vi "reference.vi"(9 "imin constant (10)":dbl=10.0 format="%.2f", 10 "GPIB":string="18") -> (0 "canceled":bool, 1 "Amax":dbl[](array[numeric])=[1.4910673946532929, 1.6585837154070626, 1.7446058754142388, 1.808885867359812, 1.8820632464916343, 1.9639766099966056, 2.0382226383687185, 2.089414045842038, 2.105029640404689, 2.0885577699852065, 2.0571333672490866, 2.027508616078245, 2.015359755409214, 2.0257112906258596, 2.0595634179012676, 2.1100473453298383, 2.172833443035523, 2.234615975589444, 2.2871273786148105, 2.3224260524059526, 2.3363376339055857, 2.331182240765136, 2.314328676539224, 2.289898733886235, 2.2678754193188975, 2.2505151462951534, 2.242292904982931, 2.24398006574108, 2.2563785464280435, 2.27769858497494, 2.3057403402615764, 2.3370197526004075, 2.366945663852573, 2.3897701311083424, 2.4032921451582543, 2.40229406080999, 2.3862474121289834, 2.3547632303177037, 2.315886415708487, 2.2697907104438184, 2.2262905051834165, 2.187520720836463, 2.160711571967675, 2.14674801363064, 2.144452774972763, 2.153387979331808, 2.171612381536747, 2.1975010961432586, 2.2293259691913074, 2.2656195831538843, 2.3051814883832087, 2.3454913564746462, 2.3821233506183246, 2.4127964287165433, 2.4358762045887516, 2.4497868469857735, 2.4546009770977615, 2.4515101179343155, 2.4418223425174155, 2.426641367561445, 2.406916405977408, 2.3842458578199786, 2.362557866554489, 2.33933415602267, 2.3189810644947233, 2.300073495267144, 2.2845660772669736, 2.2714233677435813, 2.26150315158433, 2.253967663414962, 2.2510539021873077, 2.2506151469906333, 2.2525617862063294, 2.2579664095081773, 2.2654805602840473, 2.2745273043960443, 2.28510928212571, 2.296358004741391, 2.309161557904644, 2.3221779313849757, 2.3315082762863897, 2.3426595041391187, 2.3506375453397452, 2.3588101724585626, 2.3636890556226735, 2.3664229572259727, 2.3670948931236584, 2.333326340403454, 2.224794544652323, 2.280031744138702, 2.2816718335664525, 2.270259475526624, 2.26226356693396, 2.2632572270140665, 2.2654310668267126, 2.271051261492347, 2.252318932941653, 2.2465502794425976, 2.235677394469935, 2.249345136353329, 2.2270635923428257, 2.230806428468883, 2.249200804113696, 2.2253609803726593, 2.2477278329097232, 2.2421934558224543, 2.21325471004923, 2.213995616368085, 2.2355284469075487, 2.1967287226232872, 2.2059618230596336, 2.2089248310802643, 2.233455559096529, 2.2098365950696555, 2.2121876044039577, 2.229118455328952, 2.297850204978715, 2.290123688274307, 2.251689310911409, 2.2801228963023075, 2.315594633653461, 2.2778841422402, 2.2936276917660194, 2.281533313857376, 2.293232136279035, 2.298328988073495, 2.3684356541018055, 2.3648510520076926, 2.362067585727399, 2.3472128864048627, 2.344902908055406, 2.322053817695566, 2.3018977171952084, 2.309502414966703, 2.341238602698547, 2.3314272965207428, 2.281081114278017, 2.3288686738529263, 2.336181456081918, 2.261833620575751, 2.183215731491115, 2.177997963096566, 2.21197440141396, 2.212879792163401, 2.195456833628169, 2.2016155823139427, 2.2219355998280053, 2.2220918864542596, 2.5689054149828787, 2.208387603795154, 2.1666106622894317, 2.126780577012009, 2.1150777166595804, 2.0993352776859577, 2.0773679052841567, 2.090610707828407, 2.0946108630321367, 2.0626571802255635, 2.043283665570575, 2.006123606211854, 1.9866821797795053, 1.9793662423961613, 1.9486134383505207, 1.9236584217933062, 1.8991636414772188, 1.8864907251724818, 1.852601969338235, 1.847449262499173, 1.8450980400142565, 1.8481891169913987, 1.8517535290295353, 1.843730965112092, 1.9172954009456893, 1.8857003801283296, 1.9035240644712623, 1.9124293202224247, 1.9338970927268733, 1.9433955765089543, 1.9029813997975025, 1.975059396468232, 1.902764143924086, 1.9264402033377668, 1.9214835839687896, 1.9399184203690565, 1.905364068766892, 1.9486085498764363, 1.959608944863131, 1.9838967913263057, 2.00337435401975, 2.1681437754959583, 2.370476079544294, 2.434505032502073, 2.513031053176271, 2.501251021855857, 2.6030360562505215, 2.553057325316767, 2.6755217206077972, 2.4904080015060113, 2.5658950220301104, 2.566814463504501, 2.4194286609338724, 2.452277233126352, 2.549567233145539, 2.489508491577916, 2.466036775232349, 2.5291222348209623, 2.5165882528051435, 2.5152378253184304, 2.2831654904677503, 2.1027766148834415, 2.2945103147339774, 2.278296208091274, 2.2947747522184434, 2.257102332659164, 2.1926232000129464, 2.1866738674997452, 2.1486674240110664, 2.1793794178817567, 2.081707270097349, 2.0340666785975605, 2.017705140697976, 1.918240090221415, 1.8567288903828827, 1.8983960459300089, 1.8564872128686305, 1.803320523578754, 1.7109631189952759, 1.7223047868743275, 1.6916207084305435, 1.770991846672562, 1.8018220229225788, 1.8637985386805003, 1.6497241859295224, 2.4798055677093918, 1.8810421081934057, 1.9936125579388904, 1.7551198989199506, 1.6860908247574418, 1.670255132771604, 1.6022662322285295, 1.646207612206685, 1.8161086707399037, 1.682686478249768, 1.6551384348113822, 1.732562619289829, 1.8138477542288545, 1.7537438789213702, 1.8034571156484138, 1.9565573917856787, 1.8325089127062364, 1.7867514221455612, 1.8590181438888942, 1.8106289836371174, 1.7455432019980242, 1.8923172607224805, 1.7453871213200087, 1.7158362751649936, 1.717670503002262, 1.681612038904928, 1.9141315126308938, 1.7541877393996606, 1.72965066833592, 1.8286598965353196, 1.793923026734563, 1.7128264134251168, 1.777716738609626, 1.7576996250877386, 1.7315887651867385, 1.8689969024871353, 1.8407332346118066, 1.8972971220594963, 1.9706257766882944, 1.9689496809813425, 1.9907826918031377, 1.9205407165024797, 1.9384196457931928, 1.8095597146352675, 1.7610252517113727, 1.7540423867854362, 1.823474229170301, 1.8949858218973574, 1.9153998352122696, 1.9240724299103626, 1.9669860251179379, 2.1140101617034617, 2.0889825806046582, 2.0437590536641457, 2.011316643366872, 2.049838000622583, 1.8634418286137089, 2.044069150468914, 1.9808211666443354, 1.8472023639809236, 1.721645766289746, 1.7299742856995555, 1.8672317145188941, 1.8999298827278643, 1.8678209080455728, 1.7734865759276401, 1.8046845149069402, 1.8242625467907634, 1.7199938263676038, 1.789150434745198, 1.8715729355458788, 1.6698652146556314, 1.6812412373755872, 1.665027217492617, 1.6261349786353885, 1.6803355134145632, 1.7762652182681096, 1.6748611407378116, 1.578180609627778, 1.5795549604009986, 1.611925011653304, 1.54282542695918, 1.5206145218782359] format="%.2f", 2 "IR":dbl[](array[numeric])=[309.78999999999996, 455.5999999999999, 555.4000000000001, 644.0, 762.19, 920.3999999999999, 1092.0, 1228.6100000000001, 1273.5900000000001, 1226.19, 1140.6, 1065.39, 1036.0, 1060.99, 1147.0, 1288.3899999999999, 1488.79, 1716.3899999999999, 1936.9899999999998, 2101.0, 2169.3900000000003, 2143.79, 2062.19, 1949.3899999999999, 1853.0, 1780.3899999999999, 1747.0, 1753.8000000000002, 1804.5900000000001, 1895.3899999999999, 2021.81, 2172.8, 2327.7999999999997, 2453.41, 2531.0, 2525.19, 2433.59, 2263.41, 2069.6, 1861.19, 1683.8000000000002, 1540.0, 1447.81, 1402.0, 1394.6100000000001, 1423.6, 1484.6100000000001, 1575.8000000000002, 1695.6100000000001, 1843.4, 2019.21, 2215.6, 2410.59, 2587.0, 2728.2, 2817.0, 2848.4, 2828.2, 2765.81, 2670.8, 2552.21, 2422.4, 2304.4, 2184.41, 2084.4, 1995.6, 1925.6, 1868.1999999999998, 1826.0099999999998, 1794.6, 1782.6, 1780.8000000000002, 1788.8000000000002, 1811.1999999999998, 1842.81, 1881.6, 1928.0099999999998, 1978.6, 2037.8000000000002, 2099.8, 2145.4, 2201.2, 2242.01, 2284.6, 2310.41, 2325.0, 2328.6, 2154.4, 1678.0099999999998, 1905.6, 1912.81, 1863.1999999999998, 1829.21, 1833.4, 1842.6, 1866.6, 1787.8000000000002, 1764.21, 1720.5900000000001, 1775.6, 1686.8000000000002, 1701.4, 1775.0099999999998, 1680.1999999999998, 1769.0, 1746.6, 1634.0099999999998, 1636.8000000000002, 1720.0, 1573.0, 1606.8000000000002, 1617.8000000000002, 1711.81, 1621.1999999999998, 1630.0, 1694.8000000000002, 1985.4099999999999, 1950.4, 1785.21, 1906.0, 2068.21, 1896.1999999999998, 1966.2000000000003, 1912.1999999999998, 1964.4099999999999, 1987.6, 2335.8, 2316.6, 2301.8, 2224.4, 2212.6, 2099.2, 2004.0000000000002, 2039.4, 2194.0099999999998, 2145.0, 1910.21, 2132.4, 2168.61, 1827.4, 1524.81, 1506.6, 1629.1999999999998, 1632.6, 1568.3999999999999, 1590.8000000000002, 1667.0, 1667.6, 3706.0, 1615.8000000000002, 1467.6099999999997, 1339.0, 1303.4, 1257.0, 1195.0, 1232.0, 1243.4, 1155.1999999999998, 1104.8000000000002, 1014.2, 969.8000000000001, 953.5999999999999, 888.4099999999999, 838.8, 792.8, 770.0, 712.1999999999999, 703.8, 699.9999999999999, 705.0, 710.8100000000001, 697.8, 826.5999999999999, 768.5999999999999, 800.8000000000001, 817.3900000000001, 858.81, 877.8, 799.8, 944.19, 799.4000000000001, 844.19, 834.6099999999999, 870.8, 804.1999999999999, 888.4000000000001, 911.19, 963.5999999999999, 1007.8, 1472.8, 2346.8, 2719.6, 3258.6000000000004, 3171.3999999999996, 4009.0, 3573.2, 4737.2, 3093.2, 3680.4000000000005, 3688.2, 2626.81, 2833.2, 3544.6000000000004, 3086.8, 2924.3999999999996, 3381.6000000000004, 3285.4, 3275.2, 1919.4, 1267.0, 1970.2, 1898.0, 1971.3999999999999, 1807.6, 1558.1999999999998, 1537.0, 1408.21, 1511.4, 1207.0, 1081.6, 1041.61, 828.4000000000001, 719.0, 791.4000000000001, 718.5999999999999, 635.8, 514.0000000000001, 527.5999999999999, 491.6099999999999, 590.19, 633.6099999999999, 730.8, 446.4000000000001, 3018.6, 760.4000000000001, 985.4000000000001, 569.01, 485.3900000000001, 468.0099999999999, 400.19000000000005, 442.79999999999995, 654.8, 481.5999999999999, 452.0, 540.21, 651.4000000000001, 567.21, 636.0, 904.81, 680.0, 612.0, 722.8, 646.59, 556.5999999999999, 780.4, 556.4000000000001, 519.8, 522.0, 480.40999999999997, 820.5999999999999, 567.7900000000001, 536.5999999999999, 674.0, 622.19, 516.2099999999999, 599.4000000000001, 572.4, 539.0, 739.5999999999999, 693.0, 789.3999999999999, 934.5999999999999, 930.9999999999999, 979.0, 832.8, 867.8, 645.0, 576.8, 567.5999999999999, 666.0, 785.21, 823.0, 839.5999999999999, 926.8, 1300.2000000000003, 1227.3899999999999, 1106.0099999999998, 1026.4, 1121.6000000000001, 730.2, 1106.8, 956.8, 703.4000000000001, 526.8, 537.0, 736.5999999999999, 794.2, 737.5999999999999, 593.59, 637.8, 667.21, 524.8, 615.3900000000001, 744.0, 467.5899999999999, 480.0, 462.40999999999997, 422.79999999999995, 479.0, 597.4000000000001, 473.0, 378.5999999999999, 379.79999999999995, 409.19000000000005, 349.0, 331.5999999999999] format="%.2f", 3 "GPIB":string="18")   [LabVIEW 2015]
uses:
  measurement mode.ctl
  <vilib>/Analysis/baseanly.llb/Mean (DBL).vi
  <vilib>/Analysis/NI_AALBase.lvlib
panel:
  out "mean maximum absorbance":dbl format="%.2f"
  out "?":string="Measuring absorbance of the reference sample and the lamp intensity. This will take about 30 seconds.\n\nThis information is used to determine what absorbances can be measured accurately. High absorbance values indicate little light is reaching the diode array. An absorbance value of 3 indicates that 0.001 of the incident light reached the array. At very low light levels the detection limit of the diode array controls the accuracy of the measurement.\n\nThe ability to measure high absorbance values is determined by the intensity of the incident light (a function of the lamp) and the absorbance of the reference sample. If the reference sample absorbs a significant amount of light then it will not be possible to measure high absorbances in the samples.\n\nAbsorbance values that exceed the maximum that can be measured will be reported, but will not be used in analysis."
  in  "measurement mode":T1 {"gain" max=15}
  in  "okay":bool
  out "graph":cluster{i32, i32, dbl[]}(graph)={190, 2, []}
  # "Given the lamp intensity and the absorbance of the reference this is the maximum absorbance that can be measured accurately. If the maximum absorbance is lower than expected the lamp may be failing or the reference sample may be absorbing a lot of light."
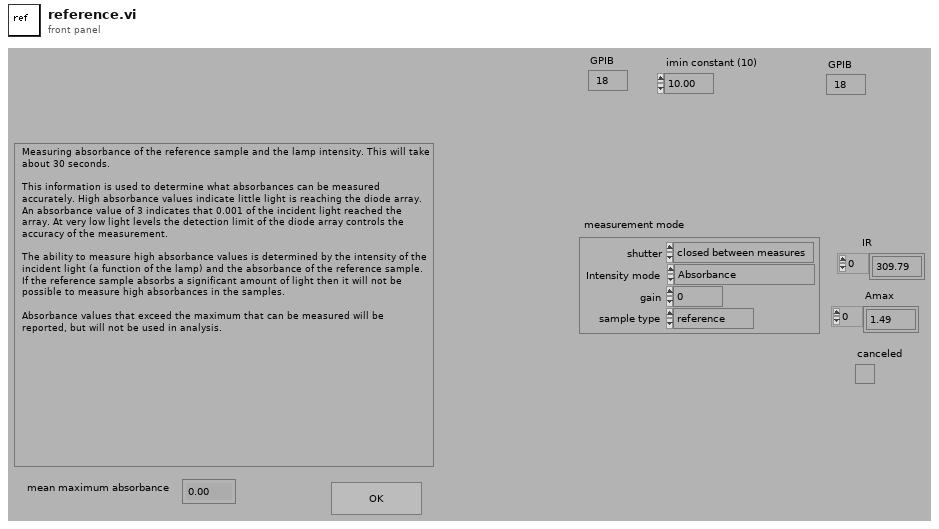
[diagram p1: front panel]
types:
  T1 = typedef "measurement mode.ctl" = cluster{"shutter":enum16{"closed between measures", "open between measures"}, "Intensity mode":enum16{"Absorbance", "Intensity at current gain", "Intensity at fixed gain", "dark current at current gain", "dark current at fixed gain"}, "gain":u8, "sample type":enum16{"reference", "standard", "unknown", "Diagnostic"}}
  T2 = typedef "settings.ctl" = cluster{"integration time":sgl, "rinse time":dbl[unit], "sample time":dbl[unit], "sample type":u16}
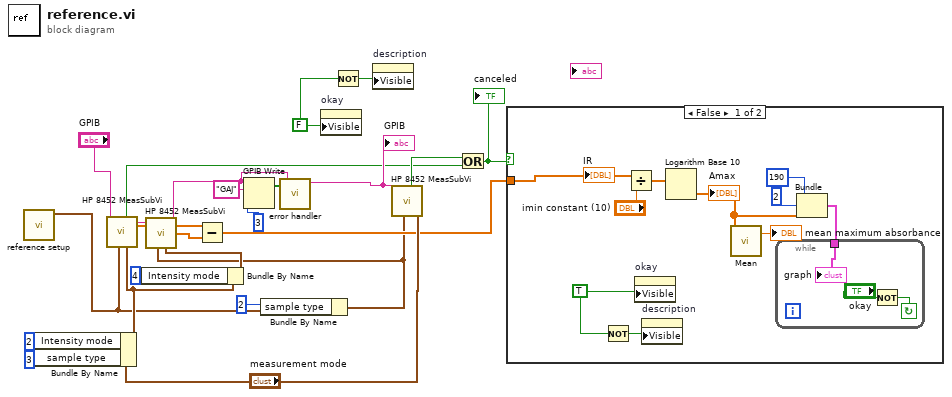
[diagram p0: block diagram]
diagram:
  w22 = FALSE
  n1 = call "reference setup.vi"() -> ("reference setup out"=w1:T2)  [unwired: 11 in]
  n2 = Bundle By Name(cluster="measurement mode", "Intensity mode"=2, "sample type"=3) -> (w8:T1)
  n3 = call "HP 8452 MeasSubVi.vi"("GPIB in"="GPIB", "setup"=w1, "measurement mode"=w8) -> ("canceled"=w14:bool, "GPIB out"=w11:string, "measurement"=w6:dbl[])  [unwired: 4 in]
  n4 = Bundle By Name(cluster=w8, "Intensity mode"=4) -> (w9:T1)
  n5 = Bundle By Name(cluster=w1, "sample type"=2) -> (w3:T2)
  n6 = call "HP 8452 MeasSubVi.vi"("GPIB in"=w11, "setup"=w3, "measurement mode"=w9) -> ("GPIB out"=w10:string, "measurement"=w5:dbl[])  [unwired: 4 in, 1 out]
  n7 = Subtract(x=w6, y=w5) -> (x-y=w4:dbl[])
  n8 = GPIB Write(0:w10, 1:"GAJ", 2:3) -> (5:w19:bool[])  [unwired: 2 in, 1 out]
  n9 = call "error handler.vi"("status array"=w19, "GPIB in"=w10) -> ("GPIB out"=w17:string)  [unwired: 3 in, 2 out]
  "GPIB" <- w17
  n10 = property on="okay" class="Bool"("Visible"=w22) -> ()  [unwired: 2 in, 2 out]
  n11 = Not(x=w22) -> (.not. x?=w21:bool)
  n12 = property on="description" class="Str"("Visible"=w21) -> ()  [unwired: 2 in, 2 out]
  n13 = call "HP 8452 MeasSubVi.vi"("GPIB in"=w17, "setup"=w3, "measurement mode"="measurement mode") -> ("canceled"=w24:bool)  [unwired: 4 in, 2 out]
  n14 = Or(x=w24, y=w14) -> (x .or. y?=w23:bool)
  "canceled" <- w23
  n15 = case shown="False" w23 {
    tunnel: w4 -> [w34 _]
    frame False {
      w28 = TRUE
      n16 = Not(x=w28) -> (.not. x?=w27:bool)
      n17 = Divide(x=w34, y="imin constant (10)") -> (x/y=w30:dbl[])
      n18 = property on="okay" class="Bool"("Visible"=w28) -> ()  [unwired: 2 in, 2 out]
      n19 = property on="description" class="Str"("Visible"=w27) -> ()  [unwired: 2 in, 2 out]
      n20 = Logarithm Base 10(1:w30) -> (0:w26:dbl[])
      "Amax" <- w26
      n21 = call-poly <vilib>:"Mean.vi"("X"=w26) -> ("mean"=→"mean maximum absorbance":dbl)  [unwired: 1 out]
      n22 = Bundle(190, 2, w26) -> (w33:cluster{i32, i32, dbl[]})  [unwired: 1 in]
      n23 = while {
        tunnel: w33 -> [w35]
        stop <- w36 continue-if-true
        n24 = Not(x="okay") -> (.not. x?=w36:bool)
        "graph" <- w35
      }
      "IR" <- w34
    }
    frame True {
    }
  }
